vi "Guess Current (N.O.).vi"(0 "input cluster":T1, 1 "VISA session":refnum<visa-resource-name>, 2 "Desired Field":dbl, 3 "Actual Field old":dbl, 4 "Current guess":dbl, 5 "error in (no error)":errorcluster, 6 "Voltage Limit":dbl=2255.0 format="%.2f", 7 "Positive?":bool) -> (14 "output cluster":T1, 15 "dup VISA session":refnum<visa-resource-name>, 16 "New guess":dbl, 18 "Stop?":bool, 19 "error out":errorcluster)   [LabVIEW 2012]
uses:
  Magna Power Constants.vi
  <vilib>/gmath/NI_Gmath.lvlib
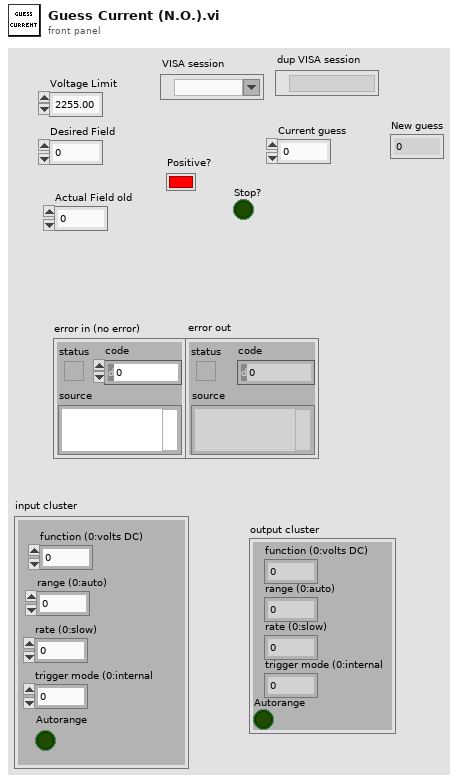
[diagram p1: front panel]
types:
  T1 = cluster{"function (0:volts DC)":i16, "range (0:auto)":i16, "rate (0:slow)":i16, "trigger mode (0:internal":i16, "Autorange":bool}
  T2 = cluster{"Field":dbl[], "Current Derivative":dbl[]}
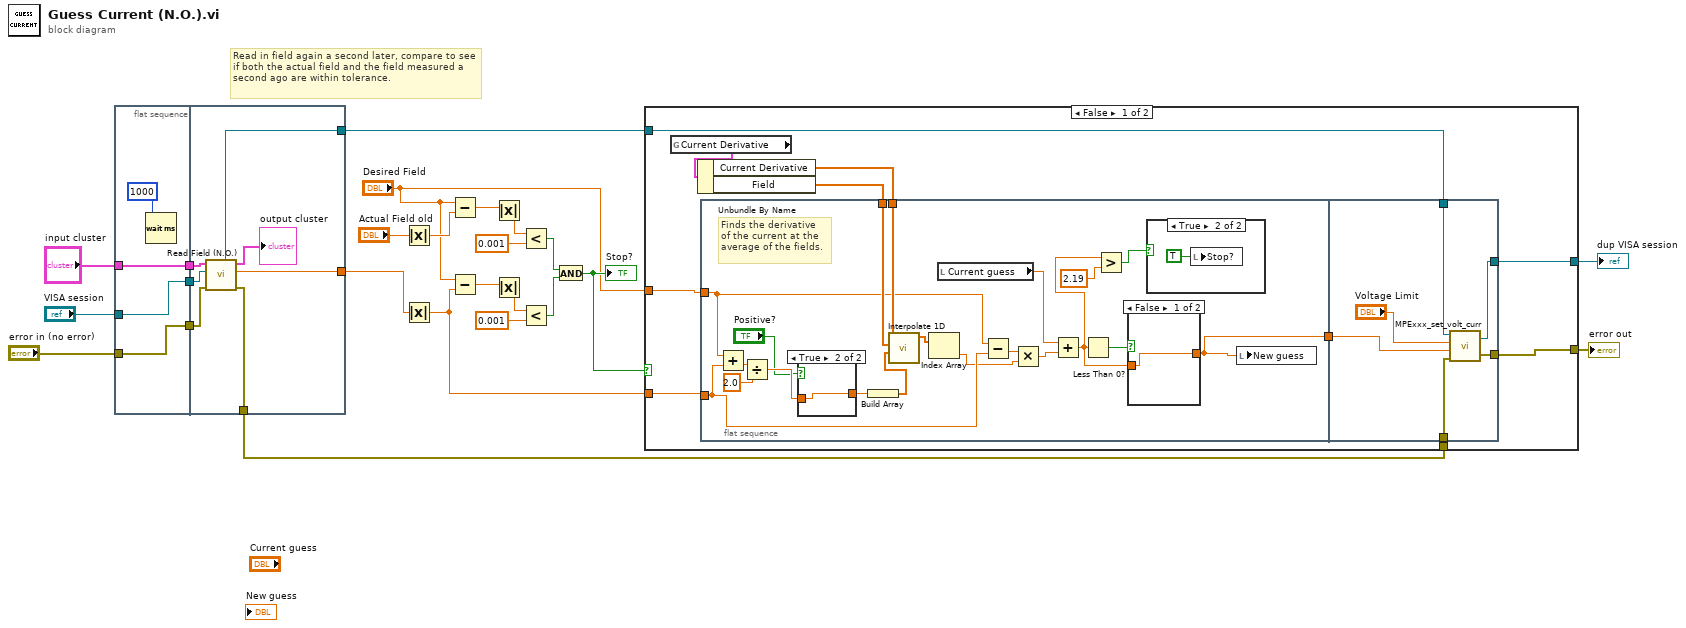
[diagram p0: block diagram]
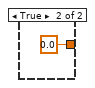
[diagram p3: hidden frame]
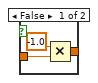
[diagram p4: hidden frame]
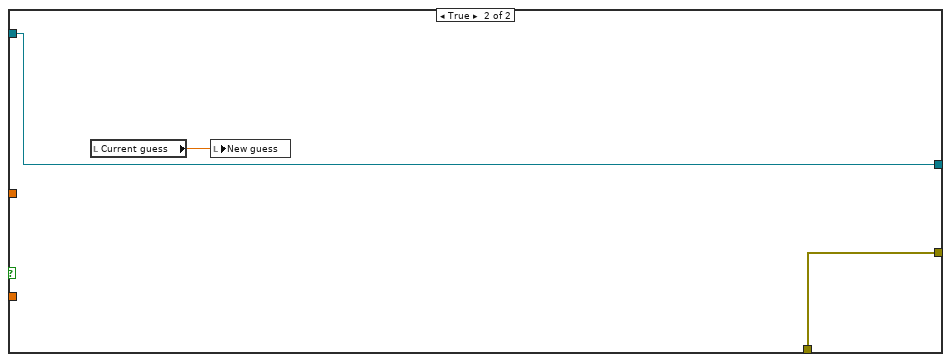
[diagram p5: hidden frame]
diagram:
  # "Read in field again a second later, compare to see if both the actual field and the field measured a second ago are within tolerance."
  n1 = flat-sequence {
    tunnel: [w27] -> w20
    tunnel: "input cluster" -> [w27]
    tunnel: [w26] -> w18
    tunnel: "VISA session" -> [w26]
    tunnel: [w25] -> w16
    tunnel: "error in (no error)" -> [w25]
    tunnel: w20 -> [w35]
    tunnel: w18 -> [w34]
    tunnel: w16 -> [w33]
    tunnel: [w31] -> w14
    tunnel: [w30] -> w13
    tunnel: [w29] -> w6
    frame #0 {
      n2 = Wait (ms)(milliseconds to wait=u32 1000) -> ()  [unwired: 1 out]
    }
    frame #1 {
      n3 = call "Read Field (N.O.).vi"("error in (no error)"=w33, "VISA session"=w34, "input cluster"=w35) -> ("error out"=w30:errorcluster, "Field (T)"=w29:dbl, "output cluster"=→"output cluster":T1, "dup VISA session"=w31:refnum<visa-resource-name>)  [unwired: 3 in, 2 out]
    }
  }
  n4 = Absolute Value(x="Actual Field old") -> (abs(x)=w12:dbl)
  n5 = Absolute Value(x=w6) -> (abs(x)=w1:dbl)
  n6 = Subtract(x="Desired Field", y=w12) -> (x-y=w11:dbl)
  n7 = Subtract(x="Desired Field", y=w1) -> (x-y=w8:dbl)
  n8 = Absolute Value(x=w11) -> (abs(x)=w10:dbl)
  n9 = Absolute Value(x=w8) -> (abs(x)=w9:dbl)
  n10 = Less?(x=w10, y=0.001) -> (x < y?=w5:bool)
  n11 = Less?(x=w9, y=0.001) -> (x < y?=w4:bool)
  n12 = And(x=w5, y=w4) -> (x .and. y?=w3:bool)
  "Stop?" <- w3
  n13 = case shown="False" w3 {
    tunnel: w13 -> [w41 w81]
    tunnel: [w40 w79] -> w24
    tunnel: [w39 w81] -> w23
    tunnel: w1 -> [w38 _]
    tunnel: "Desired Field" -> [w37 _]
    tunnel: w14 -> [w36 w79]
    frame False {
      n14 = global read "Magna Power Constants.vi" "Current Derivative"() -> (w42:T2)
      n15 = Unbundle By Name(w42) -> ("Current Derivative"=w43:dbl[], "Field"=w44:dbl[])
      n16 = flat-sequence {
        tunnel: w44 -> [w63]
        tunnel: w43 -> [w62]
        tunnel: w38 -> [w56]
        tunnel: w37 -> [w57]
        tunnel: [w51] -> w45
        tunnel: w41 -> [w78]
        tunnel: w45 -> [w75]
        tunnel: [w77] -> w39
        tunnel: [w76] -> w40
        tunnel: w36 -> [w73]
        frame #0 {
          # "Finds the derivative\nof the current at the\naverage of the fields."
          n17 = Add(x=w57, y=w56) -> (x+y=w60:dbl)
          n18 = Divide(x=w60, y=2.0) -> (x/y=w58:dbl)
          n19 = case shown="True" "Positive?" {
            tunnel: w58 -> [w70 w72]
            tunnel: [w69 w72] -> w65
            frame False {
              n20 = Multiply(x=-1.0, y=w70) -> (x*y=w69:dbl)
            }
            frame True {
            }
          }
          n21 = Build Array(w65) -> (w64:dbl[])
          n22 = call <vilib>:"Interpolate 1D.vi"("xi"=w64, "X"=w63, "Y"=w62) -> ("yi"=w61:dbl[])  [unwired: 6 in, 2 out]
          n23 = Index Array(array=w61) -> (element=w54:dbl)  [unwired: 1 in]
          n24 = local read "Current guess"() -> (w48:dbl)
          n25 = Subtract(x=w57, y=w56) -> (x-y=w55:dbl)
          n26 = Multiply(x=w55, y=w54) -> (x*y=w53:dbl)
          n27 = Add(x=w48, y=w53) -> (x+y=w46:dbl)
          n28 = Less Than 0?(x=w46) -> (x < 0?=w52:bool)
          n29 = Greater?(x=w46, y=2.19 ("x")) -> (0:w49:bool)
          n30 = case shown="False" w52 {
            tunnel: [w67 0.0] -> w51
            tunnel: w46 -> [w67 _]
            frame False {
            }
            frame True {
            }
          }
          n31 = case shown="True" w49 {
            frame False {
            }
            frame True {
              n32 = local write "Stop?"(TRUE ("Stop?")) -> ()
            }
          }
          n33 = local write "New guess"(w51) -> ()
        }
        frame #1 {
          n34 = call "MPExxx_set_volt_curr.vi"("error in (no error)"=w78, "Set Current"=w75, "Set Voltage"="Voltage Limit", "VISA session"=w73) -> ("error out"=w77:errorcluster, "dup VISA session"=w76:refnum<visa-resource-name>)
        }
      }
    }
    frame True {
      n35 = local read "Current guess"() -> (w80:dbl)
      n36 = local write "New guess"(w80) -> ()
    }
  }
  "dup VISA session" <- w24
  "error out" <- w23
